vi "RT_Read_Count_FIFO_And_Stream.vi"(8 "error in (no error)":errorcluster, 10 "Refnum in":refnum<k33>, 11 "Refnum in":refnum<k21>) -> (0 "error out":errorcluster, 2 "Network stream\n timed out":bool, 3 "endpoint out":refnum<k21>, 4 "RT FIFO errored":bool)   [LabVIEW 2020]
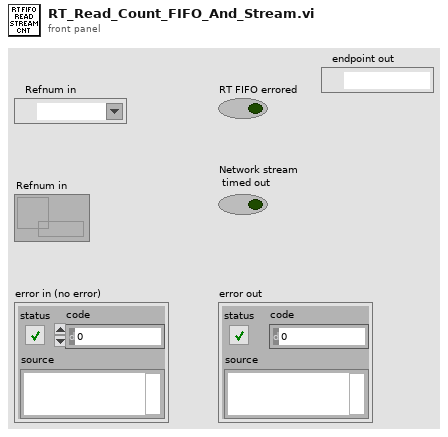
[diagram p1: front panel]
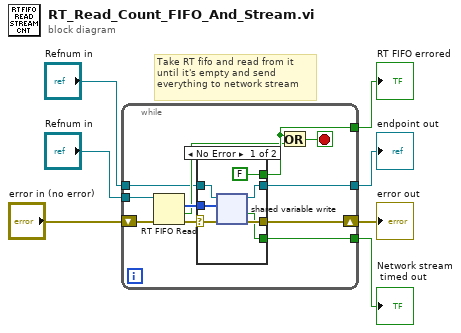
[diagram p0: block diagram]
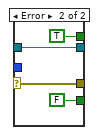
[diagram p2: hidden frame]
diagram:
  # "Take RT fifo and read from it\nuntil it's empty and send \neverything to network stream"
  n1 = while {
    tunnel: [w18] -> w2
    tunnel: "Refnum in" -> [w17]
    tunnel: "Refnum in" -> [w11]
    shift-right: [w10] -> w6
    shift-left: "error in (no error)" -> [w12]
    tunnel: [w9] -> w7
    tunnel: [w8] -> w1
    stop <- w13 stop-if-true
    n2 = RT FIFO Read(0:w17, 3:w12) -> (9:w15:i32[], 10:w14:bool, 11:w16:errorcluster)  [unwired: 2 in, 2 out]
    n3 = case shown="No Error" w16 {
      selector: w16 -> [w22 w28]
      tunnel: [FALSE TRUE] -> w18
      tunnel: w15 -> [w23 _]
      tunnel: w11 -> [w24 w26]
      tunnel: [w21 w28] -> w10
      tunnel: [w20 FALSE] -> w9
      tunnel: [w19 w26] -> w8
      frame No Error {
        n4 = shared-variable-write(w24, w22, w23) -> (w19:refnum<k21>, w21:errorcluster, w20:bool)  [unwired: 1 in]
      }
      frame Error {
      }
    }
    n5 = Or(x=w18, y=w14) -> (x .or. y?=w13:bool)
  }
  "Network stream\n timed out" <- w7
  "error out" <- w6
  "RT FIFO errored" <- w2
  "endpoint out" <- w1
